vi "LVAnalogWaveformToProtobufDoubleAnalogWaveform.vi"(8 "error in (no error)":errorcluster, 11 "Waveform":waveform(dbl)) -> (0 "error out":errorcluster, 3 "ni_protobuf_types_DoubleAnalogWaveform_Flat":T1)   [LabVIEW 2020, in "Extensions.lvlib"]
uses:
  <vilib>/gRPC/Extensions/Extensions.lvlib
  <vilib>/gRPC/Generated APIs/ni/protobuf/types/RPC Messages/ni_protobuf_types_DoubleAnalogWaveform_Flat.ctl
  <vilib>/gRPC/Generated APIs/ni/protobuf/types/RPC Messages/ni_protobuf_types_PrecisionTimestamp_Flat.ctl
  <vilib>/gRPC/Generated APIs/ni/protobuf/types/RPC Messages/ni_protobuf_types_DoubleAnalogWaveform_AttributesEntry_Flat.ctl
  <vilib>/gRPC/Generated APIs/ni/protobuf/types/RPC Messages/ni_protobuf_types_WaveformAttributeValue_Flat.ctl
  <vilib>/gRPC/Generated APIs/ni/protobuf/types/ni.protobuf.types.lvlib
  <vilib>/Utility/Data Type/NI_Data Type.lvlib
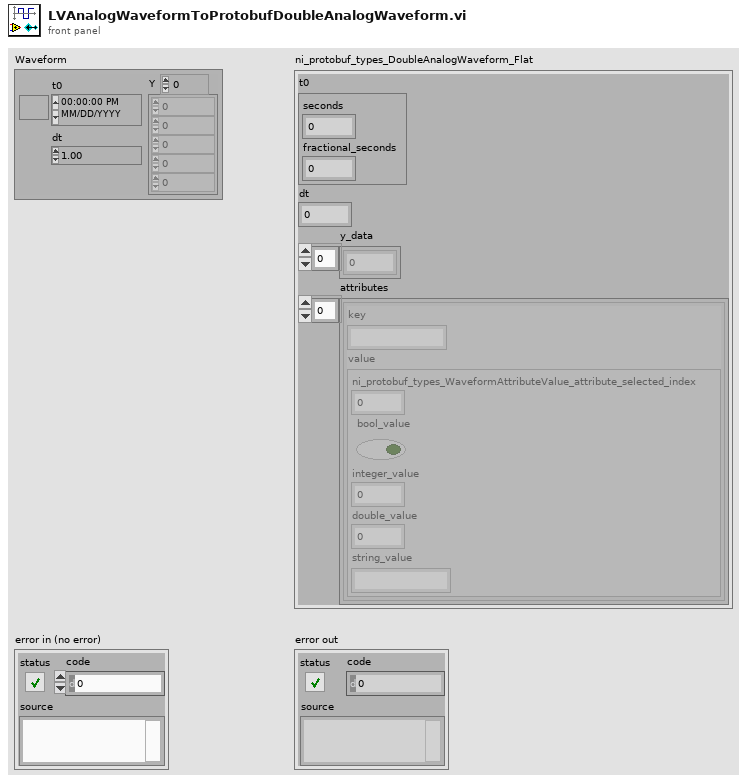
[diagram p1: front panel]
types:
  T1 = typedef "ni.protobuf.types.lvlib/ni_protobuf_types_DoubleAnalogWaveform_Flat.ctl" = cluster{"t0":T2, "dt":dbl, "y_data":dbl[], "attributes":T3[]}
  T2 = typedef "ni.protobuf.types.lvlib/ni_protobuf_types_PrecisionTimestamp_Flat.ctl" = cluster{"seconds":i64, "fractional_seconds":u64}
  T3 = typedef "ni.protobuf.types.lvlib/ni_protobuf_types_DoubleAnalogWaveform_AttributesEntry_Flat.ctl" = cluster{"key":string, "value":T4}
  T4 = typedef "ni.protobuf.types.lvlib/ni_protobuf_types_WaveformAttributeValue_Flat.ctl" = cluster{"ni_protobuf_types_WaveformAttributeValue_attribute_selected_index":i32, "bool_value":bool, "integer_value":i32, "double_value":dbl, "string_value":string}
  T5 = typedef "NI_Data Type.lvlib/Data Type.ctl" = enum8{"Invalid Type", "Void", "I8", "I16", "I32", "I64", "U8", "U16", "U32", "U64", "Single Float", "Double Float", "Extended Float", "Single Complex", "Double Complex", "Extended Complex", "Enum U8", "Enum U16", "Enum U32", "Enum U64", "Single Float With Unit", "Double Float With Unit", "Extended Float With Unit", "Single Complex with Unit", "Double Complex with Unit", "Extended Complex with Unit", "Boolean", "String", "Path", "Picture", "Tag", "Array", "Cluster", "Variant", "LV Variant", "Waveform", "Timestamp", "Digital Waveform", "Digital Data", "ExpressData", "Refnum", "External Data", "VI", "Poly VI", "LabVIEW Class Instance", "Fixed Point", "Set Collection", "Map Collection"}
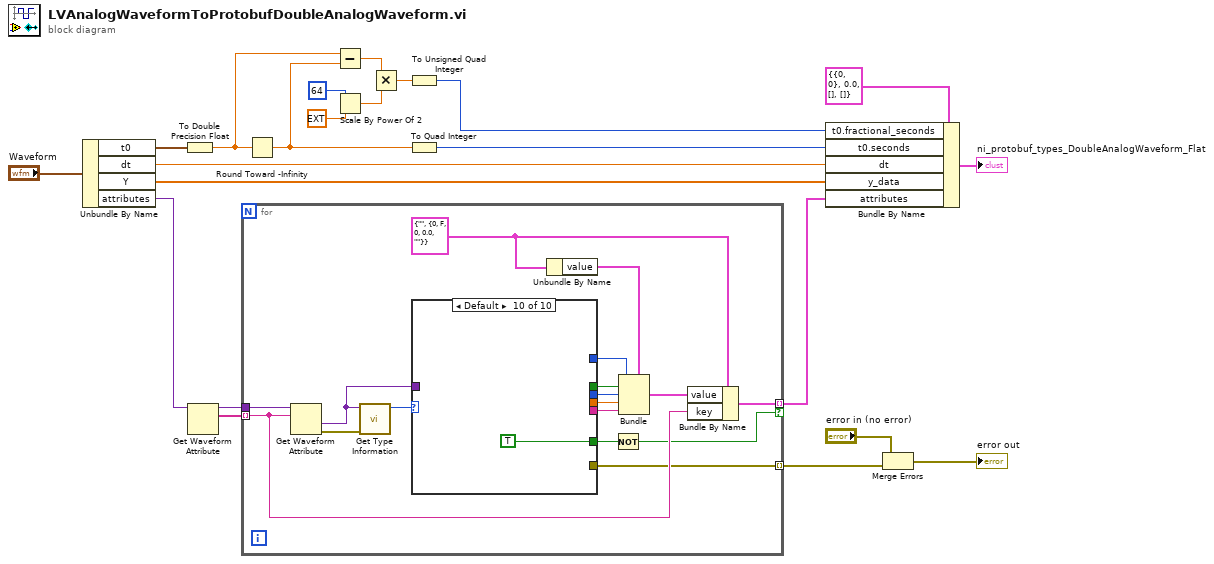
[diagram p0: block diagram]
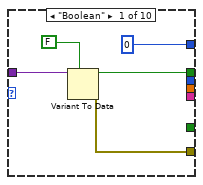
[diagram p2: hidden frame]
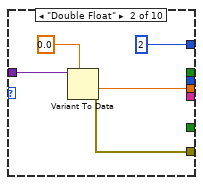
[diagram p3: hidden frame]
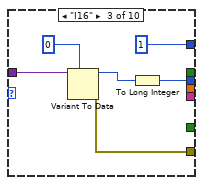
[diagram p4: hidden frame]
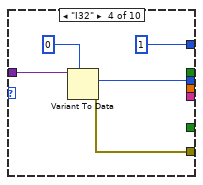
[diagram p5: hidden frame]
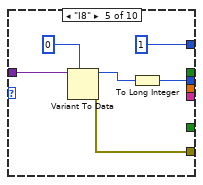
[diagram p6: hidden frame]
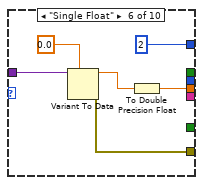
[diagram p7: hidden frame]
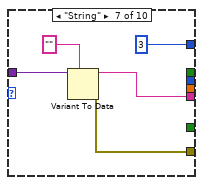
[diagram p8: hidden frame]
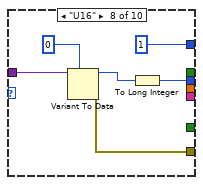
[diagram p9: hidden frame]
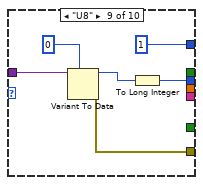
[diagram p10: hidden frame]
diagram:
  n1 = Unbundle By Name("Waveform") -> ("t0"=w13:timestamp, "dt"=w20:dbl, "Y"=w19:dbl[], "attributes"=w17:variant)
  n2 = To Double Precision Float(number=w13) -> (double precision float=w11:dbl)
  n3 = Get Waveform Attribute(7:w17) -> (2:w16:string[], 3:w15:variant)  [unwired: 3 in, 2 out]
  n4 = for {
    tunnel: w16 -> [w26] mode=indexing
    tunnel: w15 -> [w39]
    tunnel: [w27] -> w14 mode=indexing if=w23
    tunnel: [w24] -> w2 mode=indexing
    w37 = T3 {"key"="", "value"={"ni_protobuf_types_WaveformAttributeValue_attribute_selected_index"=0, "bool_value"=FALSE, "integer_value"=0, "double_value"=0.0, "string_value"=""}} ("ni_protobuf_types_DoubleAnalogWaveform_AttributesEntry_Flat")
    n5 = Get Waveform Attribute(6:w26, 7:w39) -> (0:w38:errorcluster, 1:w34:variant)  [unwired: 2 in, 2 out]
    n6 = call <vilib>:"Get Type Information.vi"("error in (no error)"=w38, "variant"=w34) -> ("type"=w35:T5)  [unwired: 5 in, 4 out]
    n7 = case shown="Default" w35 {
      tunnel: w34 -> [w44 w49 w55 w60 w66 w72 w77 w83 w89 _]
      tunnel: [w42 _ _ _ _ _ _ _ _ _] -> w33
      tunnel: [0 2 1 1 1 2 3 1 1 _] -> w32
      tunnel: [_ _ w52 w57 w63 _ _ w80 w86 _] -> w31
      tunnel: [_ w46 _ _ _ w68 _ _ _ _] -> w30
      tunnel: [_ _ _ _ _ _ w74 _ _ _] -> w29
      tunnel: [_ _ _ _ _ _ _ _ _ TRUE] -> w25
      tunnel: [w40 w45 w50 w56 w61 w67 w73 w78 w84 _] -> w24
      frame "Boolean" {
        n8 = Variant To Data(type=FALSE, Variant=w44) -> (data=w42:bool, error out=w40:errorcluster)  [unwired: 1 in]
      }
      frame "Double Float" {
        n9 = Variant To Data(type=0.0, Variant=w49) -> (data=w46:dbl, error out=w45:errorcluster)  [unwired: 1 in]
      }
      frame "I16" {
        n10 = Variant To Data(type=i16 0, Variant=w55) -> (data=w51:i16, error out=w50:errorcluster)  [unwired: 1 in]
        n11 = To Long Integer(number=w51) -> (32bit integer=w52:i32)
      }
      frame "I32" {
        n12 = Variant To Data(type=0, Variant=w60) -> (data=w57:i32, error out=w56:errorcluster)  [unwired: 1 in]
      }
      frame "I8" {
        n13 = Variant To Data(type=i8 0, Variant=w66) -> (data=w62:i8, error out=w61:errorcluster)  [unwired: 1 in]
        n14 = To Long Integer(number=w62) -> (32bit integer=w63:i32)
      }
      frame "Single Float" {
        n15 = Variant To Data(type=sgl 0.0, Variant=w72) -> (data=w69:sgl, error out=w67:errorcluster)  [unwired: 1 in]
        n16 = To Double Precision Float(number=w69) -> (double precision float=w68:dbl)
      }
      frame "String" {
        n17 = Variant To Data(type="", Variant=w77) -> (data=w74:string, error out=w73:errorcluster)  [unwired: 1 in]
      }
      frame "U16" {
        n18 = Variant To Data(type=u16 0, Variant=w83) -> (data=w79:u16, error out=w78:errorcluster)  [unwired: 1 in]
        n19 = To Long Integer(number=w79) -> (32bit integer=w80:i32)
      }
      frame "U8" {
        n20 = Variant To Data(type=u8 0, Variant=w89) -> (data=w85:u8, error out=w84:errorcluster)  [unwired: 1 in]
        n21 = To Long Integer(number=w85) -> (32bit integer=w86:i32)
      }
      frame Default {
      }
    }
    n22 = Unbundle By Name(w37) -> ("value"=w36:T4)
    n23 = Not(x=w25) -> (.not. x?=w23:bool)
    n24 = Bundle(cluster=w36, "ni_protobuf_types_WaveformAttributeValue_attribute_selected_index"=w32, "bool_value"=w33, "integer_value"=w31, "double_value"=w30, "string_value"=w29) -> (w28:T4)
    n25 = Bundle By Name(cluster=w37, "value"=w28, "key"=w26) -> (w27:T3)
  }
  n26 = Round Toward -Infinity(1:w11) -> (0:w10:dbl)
  n27 = Subtract(x=w11, y=w10) -> (x-y=w9:dbl)
  n28 = Scale By Power Of 2(n=i16 64, x=ext 1.0) -> (x*2^n=w6:ext)
  n29 = Multiply(x=w9, y=w6) -> (x*y=w5:ext)
  n30 = To Unsigned Quad Integer(1:w5) -> (0:w4:u64)
  n31 = To Quad Integer(1:w10) -> (0:w12:i64)
  n32 = Bundle By Name(cluster=T1 {"t0"={"seconds"=0, "fractional_seconds"=0}, "dt"=0.0, "y_data"=[], "attributes"=[]} ("ni_protobuf_types_DoubleAnalogWaveform_Flat"), "t0.fractional_seconds"=w4, "t0.seconds"=w12, "dt"=w20, "y_data"=w19, "attributes"=w14) -> (→"ni_protobuf_types_DoubleAnalogWaveform_Flat":T1)
  n33 = Merge Errors("error in (no error)", w2) -> (→"error out":errorcluster)
